vi "EnumExample.vi"() -> ()   [LabVIEW 2020]
panel:
  out "Status":string
  in  "stop":bool
  in  "enum":i32(ring) items=["Add item ...", "new item000", "new item001"]
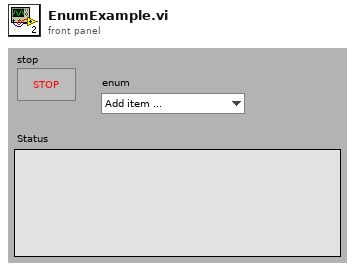
[diagram p1: front panel]
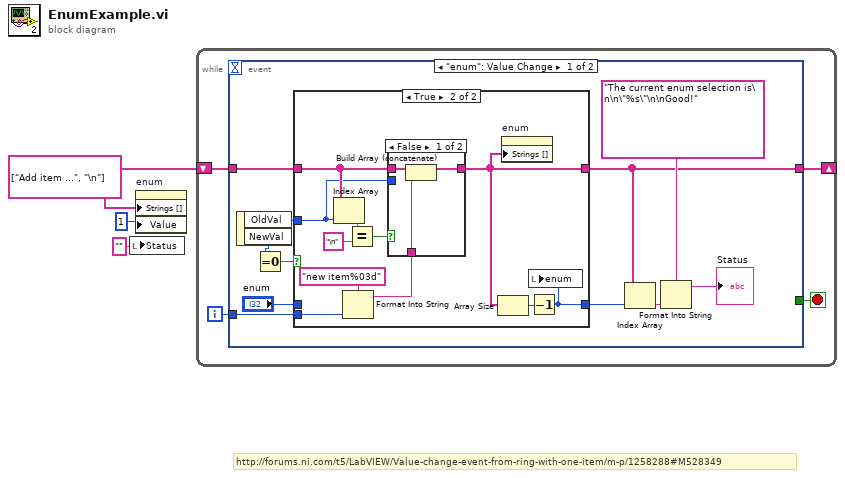
[diagram p0: block diagram]
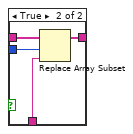
[diagram p3: hidden frame]
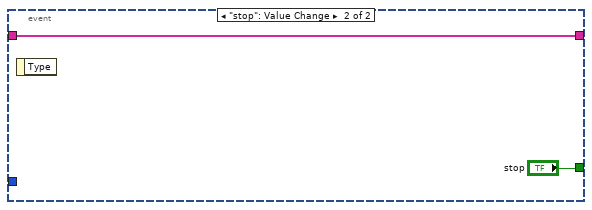
[diagram p4: hidden frame]
diagram:
  w3 = string[] ["Add item ...", "\n"] ("Strings []")
  # "http://forums.ni.com/t5/LabVIEW/Value-change-event-from-ring-with-one-item/m-p/1258288#M528349"
  n1 = local write "Status"("" ("Status")) -> ()
  n2 = property on="enum" class="Ring (strict)"("Strings []"=w3, "Value"=1) -> ()  [unwired: 2 in, 2 out]
  n3 = while {
    shift-right: [w5] -> _
    shift-left: w3 -> [w6]
    i -> [w4]
    stop <- w7 stop-if-true
    n4 = event shown="[0] \"enum\": Value Change" {
      selector: _ -> [_ _]
      dyn-events: _ -> [_ _]
      timeout: _ -> [_ _]
      tunnel: [_ "stop"] -> w7
      tunnel: w6 -> [w14 w39]
      tunnel: [w13 w39] -> w5
      tunnel: w4 -> [w8 _]
      event "enum": Value Change {
        n5 = event-data() -> ("OldVal"=w12:i32, "NewVal"=w15:i32)  [unwired: 1 in]
        n6 = Equal To 0?(x=w15) -> (x = 0?=w11:bool)
        n7 = case shown="True" w11 {
          tunnel: w14 -> [w20 w27]
          tunnel: [w20 w21] -> w13
          tunnel: w12 -> [_ w26]
          tunnel: [w19 w28] -> w10
          tunnel: "enum" -> [w19 _]
          tunnel: w8 -> [_ w30]
          frame False {
          }
          frame True {
            n8 = Index Array(array=w27, index=w26) -> (element=w25:string)
            n9 = Format Into String(format string="new item%03d", w30) -> (resulting string=w22:string)  [unwired: 2 in, 1 out]
            n10 = Equal?(x=w25, y="\n") -> (x = y?=w24:bool)
            n11 = case shown="False" w24 {
              tunnel: w27 -> [w34 w38]
              tunnel: [w33 w37] -> w21
              tunnel: w26 -> [_ w36]
              tunnel: w22 -> [w32 w35]
              frame False {
                n12 = Build Array (concatenate)(w34, w32) -> (w33:string[])
              }
              frame True {
                n13 = Replace Array Subset(array=w38, new element=w35, index=w36) -> (w37:string[])
              }
            }
            n14 = Array Size(array=w21) -> (size(s)=w29:i32)
            n15 = property on="enum" class="Ring (strict)"("Strings []"=w21) -> ()  [unwired: 2 in, 2 out]
            n16 = Decrement(x=w29) -> (x-1=w28:i32)
            n17 = local write "enum"(w28) -> ()
          }
        }
        n18 = Index Array(array=w13, index=w10) -> (element=w18:string)
        n19 = Format Into String(format string="The current enum selection is\n\n\"%s\"\n\nGood!", w18) -> (resulting string=→"Status":string)  [unwired: 2 in, 1 out]
      }
      event "stop": Value Change {
        n20 = event-data() -> ()  [unwired: 1 in, 1 out]
      }
    }
  }
